vi "PID_controller_07.vi"() -> ()   [LabVIEW 2011]
uses:
  <vilib>/Platform/TimedLoop/XDataNode/nitl_modes.ctl
  <vilib>/Platform/TimedLoop/XDataNode/timing_clust.ctl
  <vilib>/Platform/TimedLoop/XDataNode/wakeup.ctl
  <vilib>/Platform/TimedLoop/XDataNode/XDataNode.xnode
  <vilib>/Platform/TimedLoop/XDataNode/XDNodeRunTimeDep.lvlib
panel:
  in  "Ks":dbl
  out "dt(s)":dbl
  out "windup error":dbl
  out "tPrev":dbl
  out "calc value":dbl
  out "error(t-t0)":cluster{dbl, "Value":dbl}[](array[cluster])
  out "error":dbl
  out "tStart(s)":dbl
  out "x-y":dbl
  out "S00":dbl
  out "S10":dbl
  out "S20":dbl
  out "S11":dbl
  out "S01":dbl
  out "weight":dbl[](array[numeric])
  in  "# of points to watch":i32
  in  "tSmooth(s)":dbl=-1.0
  out "t0":dbl
  out "error(t)":cluster{dbl, "Value":dbl}[](array[cluster])
  out "error out":errorcluster
  out "first":bool=TRUE
  out "P (torr)":string
  out "XY Graph":cluster{dbl, "Value":dbl}[](graph)
  out "current value":dbl
  in  "stop":bool
  in  "Period (s)":dbl
  out "dValue":dbl
  out "derivative":dbl
  out "integral":dbl
  out "Current angle (deg)":dbl
  in  "Kd":dbl
  in  "Ki":dbl
  in  "Kp":dbl
  out "Current P (torr)":dbl
  in  "Set Point (torr)":dbl
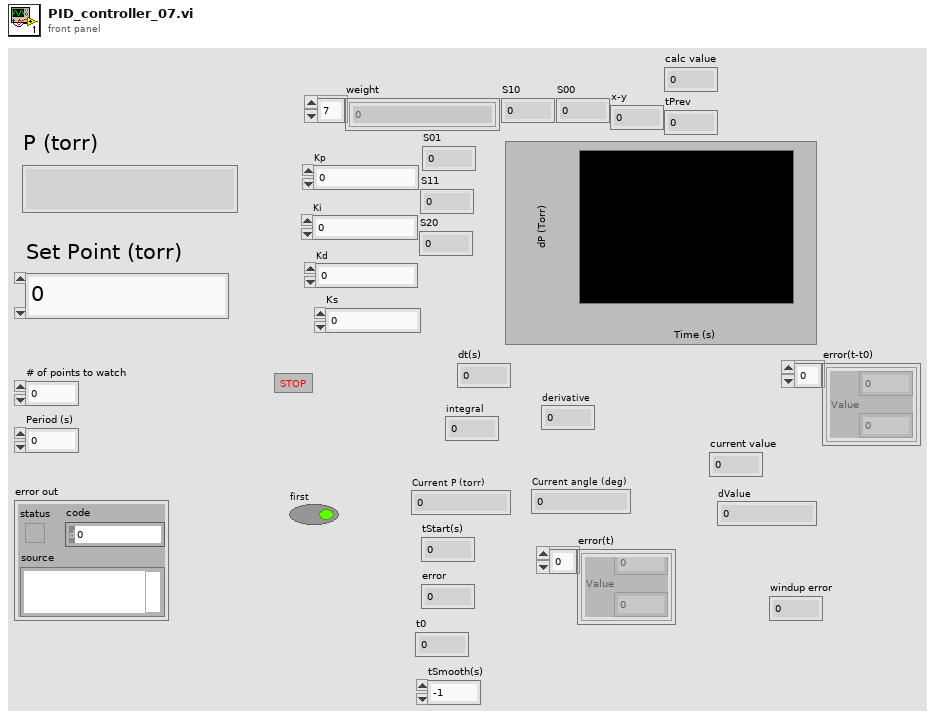
[diagram p1: front panel]
types:
  T1 = typedef "XDNodeRunTimeDep.lvlib/nitl_modes.ctl" = enum32{"No Change", "Process missed periods, maintain original phase", "Discard missed periods, maintain original phase", "Process missed periods, ignore original phase", "Discard missed periods, ignore original phase"}
  T2 = typedef "XDNodeRunTimeDep.lvlib/timing_clust.ctl" = cluster{"Expected End [f-1]":u64, "Actual End [f-1]":u64, "Finished Late? [f-1]":bool, "Expected End [i-1]":u64, "Actual End [i-1]":u64, "Finished Late? [i-1]":bool, "Expected Start [i]":u64, "Actual Start [i]":u64, "Expected Start [f]":u64, "Actual Start [f]":u64, "Source Name":string, "Structure Name":string, "Period":i64, "Deadline":i64, "Offset":i64, "Start":i64, "Priority":i32, "Timeout":i32, "Mode":T1, "Wakeup Reason":T3, "Error":errorcluster, "Source Type":string, "Secondary Source Type":string, "Global End Time":u64, "Global Start Time":u64, "Frame Duration":u64, "Iteration Duration":u64, "Assigned CPU":i32, "I/O Scan Engine Mode":u32}
  T3 = typedef "XDNodeRunTimeDep.lvlib/wakeup.ctl" = enum32{"Normal", "Aborted", "Asynchronous wakeup", "Timing source error", "Timed loop error", "Timeout"}
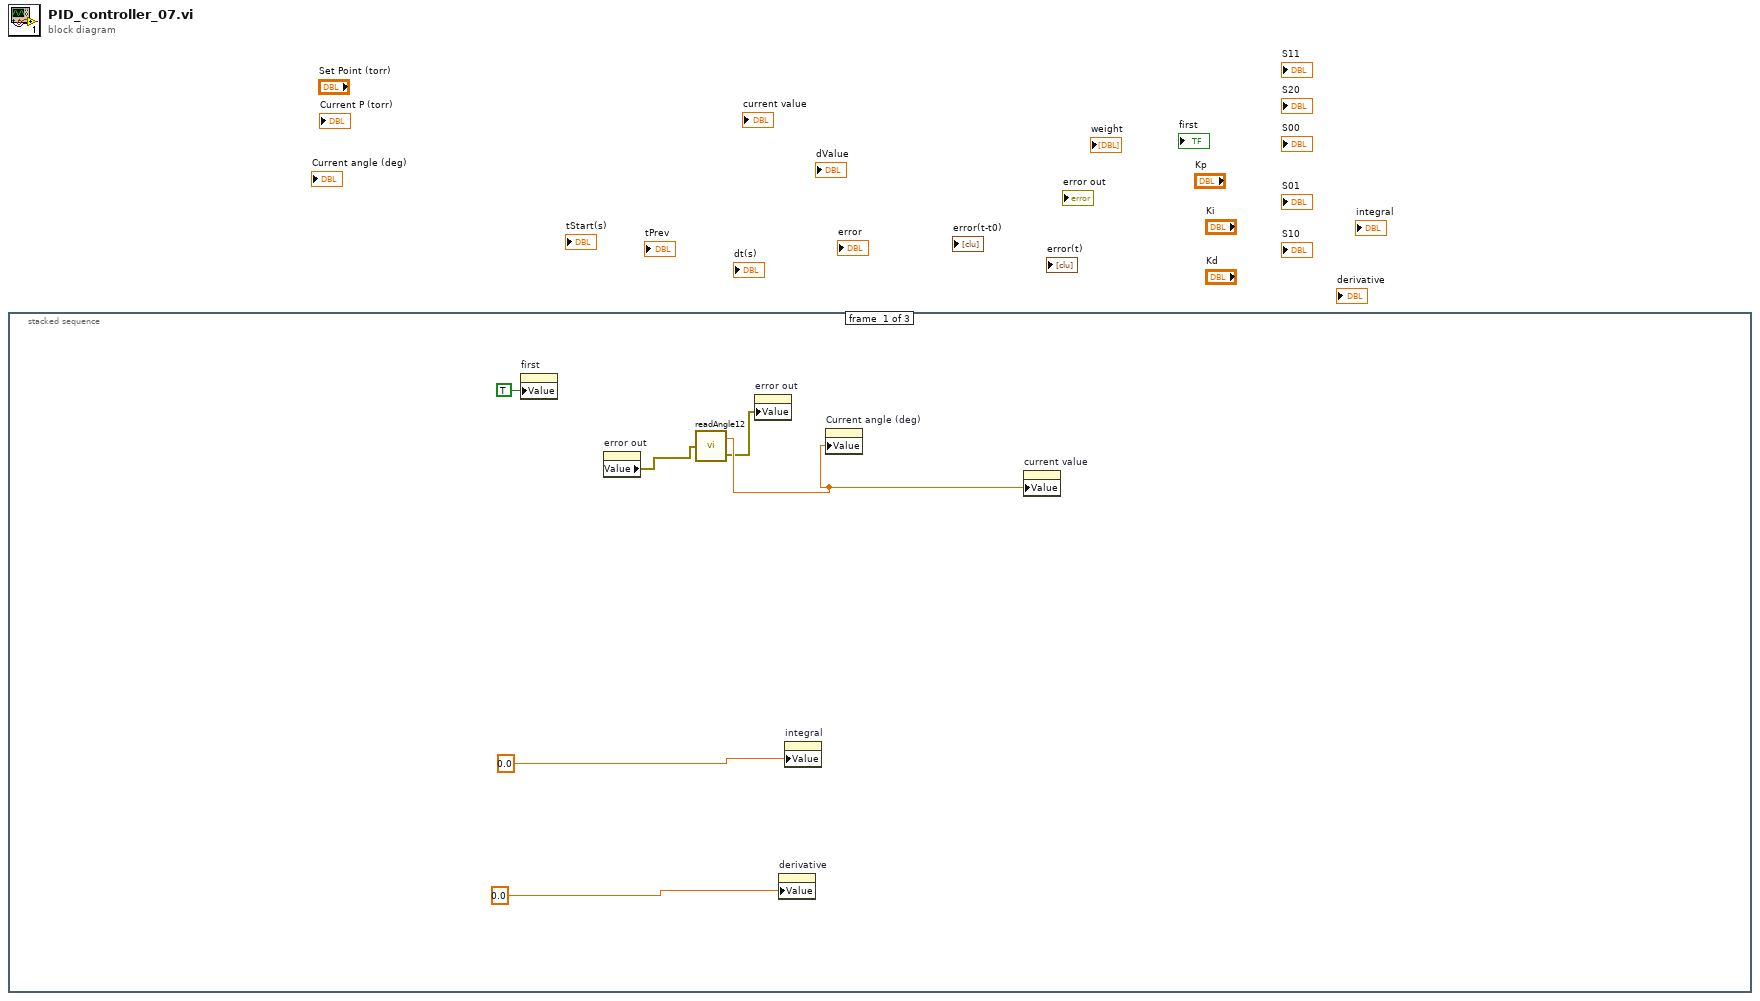
[diagram p0: block diagram]
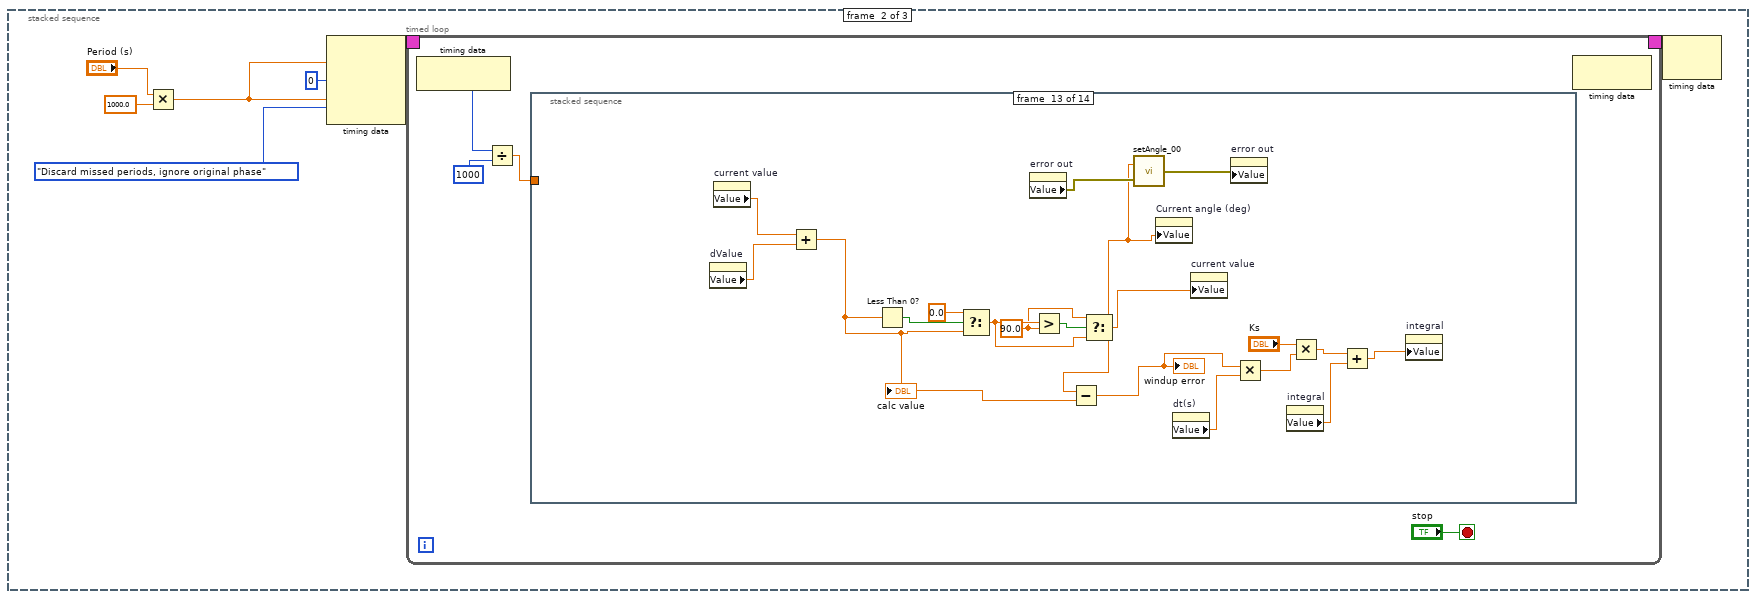
[diagram p2: hidden frame]
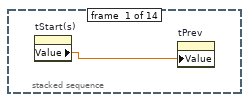
[diagram p3: hidden frame]
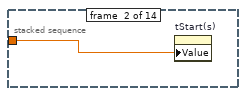
[diagram p4: hidden frame]
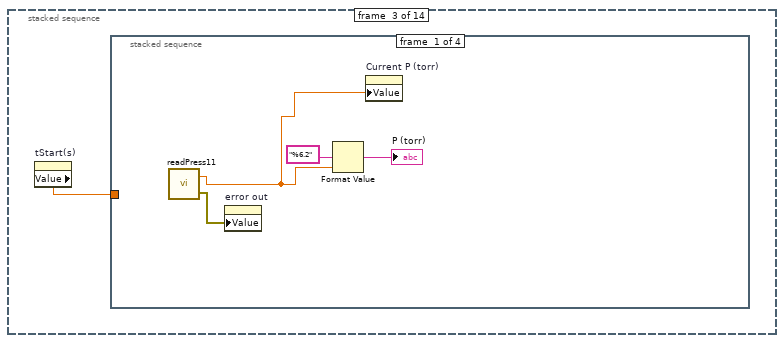
[diagram p5: hidden frame]
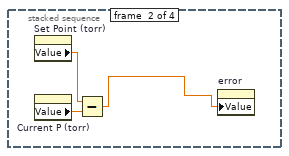
[diagram p6: hidden frame]
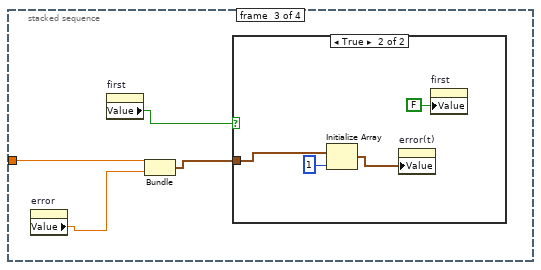
[diagram p7: hidden frame]
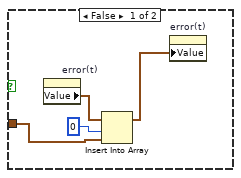
[diagram p8: hidden frame]
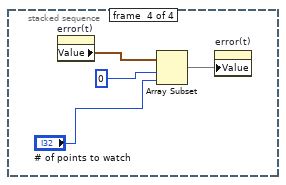
[diagram p9: hidden frame]
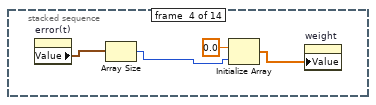
[diagram p10: hidden frame]
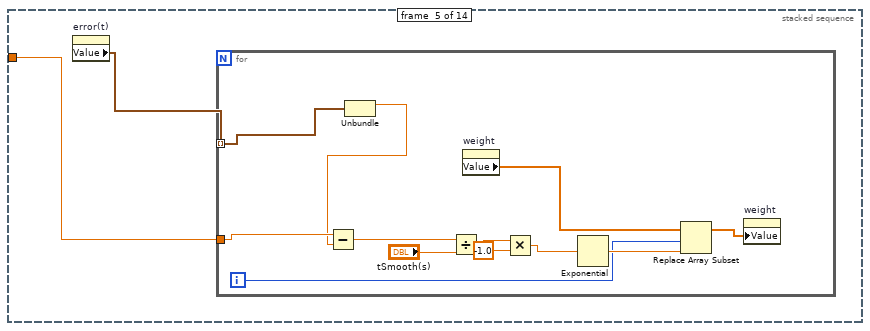
[diagram p11: hidden frame]
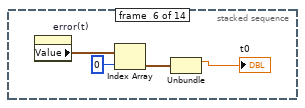
[diagram p12: hidden frame]
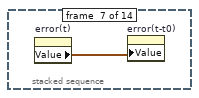
[diagram p13: hidden frame]
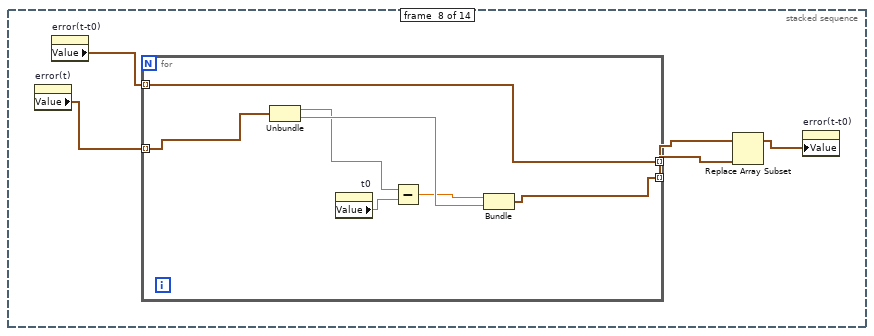
[diagram p14: hidden frame]
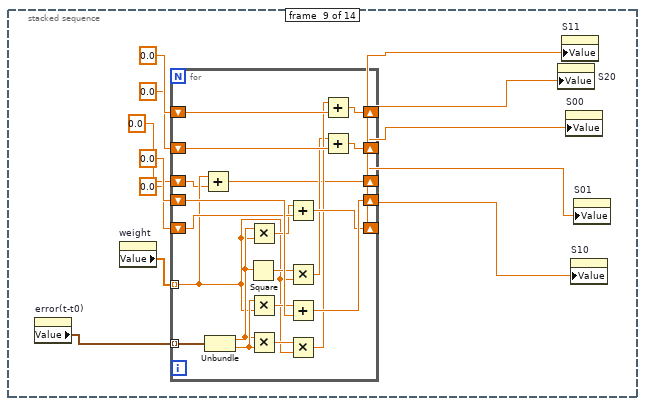
[diagram p15: hidden frame]
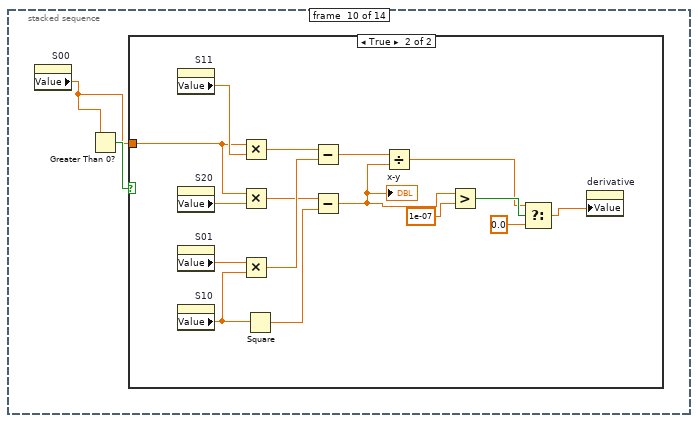
[diagram p16: hidden frame]
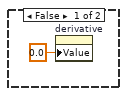
[diagram p17: hidden frame]
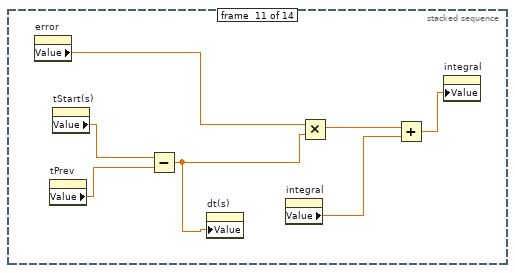
[diagram p18: hidden frame]
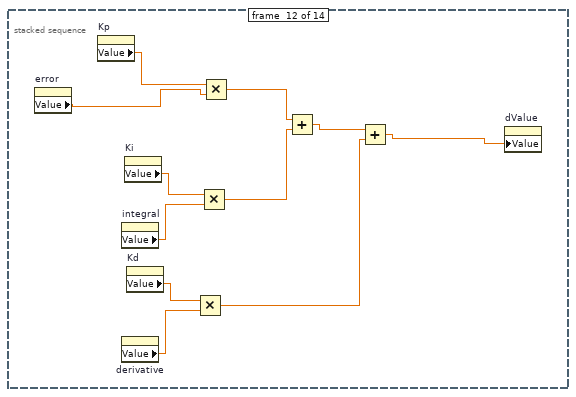
[diagram p19: hidden frame]
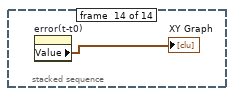
[diagram p20: hidden frame]
diagram:
  n1 = stacked-sequence {
    frame #0 {
      n2 = property on="first" class="Bool (strict)"("Value"=TRUE ("first")) -> ()  [unwired: 2 in, 2 out]
      n3 = property on="error out" class="Clust (strict)"() -> ("Value"=w2:errorcluster)  [unwired: 2 in, 2 out]
      n4 = call "readAngle12.vi"("error in"=w2) -> ("angle"=w3:dbl, "error out"=w1:errorcluster)
      n5 = property on="error out" class="Clust (strict)"("Value"=w1) -> ()  [unwired: 2 in, 2 out]
      n6 = property on="derivative" class="DigNum (strict)"("Value"=0.0 ("derivative")) -> ()  [unwired: 2 in, 2 out]
      n7 = property on="integral" class="DigNum (strict)"("Value"=0.0 ("integral")) -> ()  [unwired: 2 in, 2 out]
      n8 = property on="Current angle (deg)" class="DigNum (strict)"("Value"=w3) -> ()  [unwired: 2 in, 2 out]
      n9 = property on="current value" class="DigNum (strict)"("Value"=w3) -> ()  [unwired: 2 in, 2 out]
    }
    frame #1 {
      n10 = Multiply(x="Period (s)", y=1000.0) -> (x*y=w8:dbl)
      n11 = node-c288(w8, i64 0 ("Offset"), w8, nitl_modes."Discard missed periods, ignore original phase" ("Mode")) -> (w13:T2)
      n12 = timed-loop {
        timing: w13 -> [_]
        timing-out: [_] -> w12
        stop <- "stop" stop-if-true
        n13 = node-c288() -> (w14:i64)  [unwired: 1 in]
        n14 = Divide(x=w14, y=i64 1000) -> (x/y=w15:dbl)
        n15 = stacked-sequence {
          tunnel: w15 -> [_ w19 _ _ w48 _ _ _ _ _ _ _ _ _]
          frame #0 {
            n16 = property on="tStart(s)" class="DigNum (strict)"() -> ("Value"=w18:dbl)  [unwired: 2 in, 2 out]
            n17 = property on="tPrev" class="DigNum (strict)"("Value"=w18) -> ()  [unwired: 2 in, 2 out]
          }
          frame #1 {
            n18 = property on="tStart(s)" class="DigNum (strict)"("Value"=w19) -> ()  [unwired: 2 in, 2 out]
          }
          frame #2 {
            n19 = property on="tStart(s)" class="DigNum (strict)"() -> ("Value"=w20:dbl)  [unwired: 2 in, 2 out]
            n20 = stacked-sequence {
              tunnel: w20 -> [_ _ w30 _]
              frame #0 {
                n21 = call "readPress11.vi"() -> ("P"=w22:dbl, "error out"=w21:errorcluster)  [unwired: 1 in]
                n22 = property on="error out" class="Clust (strict)"("Value"=w21) -> ()  [unwired: 2 in, 2 out]
                n23 = Format Value(format string="%6.2", value (0)=w22) -> (output string=→"P (torr)":string)  [unwired: 1 in]
                n24 = property on="Current P (torr)" class="DigNum (strict)"("Value"=w22) -> ()  [unwired: 2 in, 2 out]
              }
              frame #1 {
                n25 = property on="Set Point (torr)" class="DigNum (strict)"() -> ("Value"=w26:dbl)  [unwired: 2 in, 2 out]
                n26 = property on="Current P (torr)" class="DigNum (strict)"() -> ("Value"=w27:dbl)  [unwired: 2 in, 2 out]
                n27 = Subtract(x=w26, y=w27) -> (x-y=w25:dbl)
                n28 = property on="error" class="DigNum (strict)"("Value"=w25) -> ()  [unwired: 2 in, 2 out]
              }
              frame #2 {
                n29 = property on="error" class="DigNum (strict)"() -> ("Value"=w28:dbl)  [unwired: 2 in, 2 out]
                n30 = property on="first" class="Bool (strict)"() -> ("Value"=w31:bool)  [unwired: 2 in, 2 out]
                n31 = Bundle("Value"=w30, "Value"=w28) -> (w29:cluster{"Value":dbl, "Value":dbl})  [unwired: 1 in]
                n32 = case shown="True" w31 {
                  tunnel: w29 -> [w33 w38]
                  frame False {
                    n33 = property on="error(t)" class="Arr (strict)"() -> ("Value"=w34:cluster{dbl, "Value":dbl}[])  [unwired: 2 in, 2 out]
                    n34 = Insert Into Array(array=w34, index=0, new element=w33) -> (w32:cluster{dbl, "Value":dbl}[])
                    n35 = property on="error(t)" class="Arr (strict)"("Value"=w32) -> ()  [unwired: 2 in, 2 out]
                  }
                  frame True {
                    n36 = Initialize Array(w38, 1 ("dimension size")) -> (w36:cluster{"Value":dbl, "Value":dbl}[])
                    n37 = property on="error(t)" class="Arr (strict)"("Value"=w36) -> ()  [unwired: 2 in, 2 out]
                    n38 = property on="first" class="Bool (strict)"("Value"=FALSE ("first")) -> ()  [unwired: 2 in, 2 out]
                  }
                }
              }
              frame #3 {
                n39 = property on="error(t)" class="Arr (strict)"() -> ("Value"=w41:cluster{dbl, "Value":dbl}[])  [unwired: 2 in, 2 out]
                n40 = Array Subset(array=w41, index=0, length="# of points to watch") -> (w43:cluster{dbl, "Value":dbl}[])
                n41 = property on="error(t)" class="Arr (strict)"("Value"=w43) -> ()  [unwired: 2 in, 2 out]
              }
            }
          }
          frame #3 {
            n42 = property on="error(t)" class="Arr (strict)"() -> ("Value"=w47:cluster{dbl, "Value":dbl}[])  [unwired: 2 in, 2 out]
            n43 = Array Size(array=w47) -> (size(s)=w45:i32)
            n44 = Initialize Array(0.0 ("element"), w45) -> (w44:dbl[])
            n45 = property on="weight" class="Arr (strict)"("Value"=w44) -> ()  [unwired: 2 in, 2 out]
          }
          frame #4 {
            n46 = property on="error(t)" class="Arr (strict)"() -> ("Value"=w49:cluster{dbl, "Value":dbl}[])  [unwired: 2 in, 2 out]
            n47 = for {
              tunnel: w49 -> [w61] mode=indexing
              tunnel: w48 -> [w60]
              i -> [w56]
              n48 = Unbundle(w61) -> (w59:dbl)  [unwired: 1 out]
              n49 = Subtract(x=w60, y=w59) -> (x-y=w54:dbl)
              n50 = Divide(x=w54, y="tSmooth(s)") -> (x/y=w52:dbl)
              n51 = property on="weight" class="Arr (strict)"() -> ("Value"=w57:dbl[])  [unwired: 2 in, 2 out]
              n52 = Multiply(x=w52, y=-1.0) -> (x*y=w50:dbl)
              n53 = Exponential(1:w50) -> (0:w58:dbl)
              n54 = Replace Array Subset(array=w57, new element=w58, index=w56) -> (w55:dbl[])
              n55 = property on="weight" class="Arr (strict)"("Value"=w55) -> ()  [unwired: 2 in, 2 out]
            }
          }
          frame #5 {
            n56 = property on="error(t)" class="Arr (strict)"() -> ("Value"=w65:cluster{dbl, "Value":dbl}[])  [unwired: 2 in, 2 out]
            n57 = Index Array(array=w65, index=0) -> (element=w63:cluster{dbl, "Value":dbl})
            n58 = Unbundle(w63) -> (→"t0":dbl)  [unwired: 1 out]
          }
          frame #6 {
            n59 = property on="error(t)" class="Arr (strict)"() -> ("Value"=w66:cluster{dbl, "Value":dbl}[])  [unwired: 2 in, 2 out]
            n60 = property on="error(t-t0)" class="Arr (strict)"("Value"=w66) -> ()  [unwired: 2 in, 2 out]
          }
          frame #7 {
            n61 = property on="error(t)" class="Arr (strict)"() -> ("Value"=w71:cluster{dbl, "Value":dbl}[])  [unwired: 2 in, 2 out]
            n62 = property on="error(t-t0)" class="Arr (strict)"() -> ("Value"=w69:cluster{dbl, "Value":dbl}[])  [unwired: 2 in, 2 out]
            n63 = for {
              tunnel: w71 -> [w74] mode=indexing
              tunnel: [w73] -> w70 mode=indexing
              tunnel: w69 -> [w72] mode=indexing
              tunnel: [w72] -> w68 mode=indexing
              n64 = Unbundle(w74) -> (w75:dbl, "Value"=w77:dbl)
              n65 = property on="t0" class="DigNum (strict)"() -> ("Value"=w78:dbl)  [unwired: 2 in, 2 out]
              n66 = Subtract(x=w75, y=w78) -> (x-y=w76:dbl)
              n67 = Bundle(w76, "Value"=w77) -> (w73:cluster{dbl, "Value":dbl})  [unwired: 1 in]
            }
            n68 = Replace Array Subset(array=w68, new element=w70) -> (w67:cluster{dbl, "Value":dbl}[])  [unwired: 1 in]
            n69 = property on="error(t-t0)" class="Arr (strict)"("Value"=w67) -> ()  [unwired: 2 in, 2 out]
          }
          frame #8 {
            n70 = property on="error(t-t0)" class="Arr (strict)"() -> ("Value"=w79:cluster{dbl, "Value":dbl}[])  [unwired: 2 in, 2 out]
            n71 = property on="weight" class="Arr (strict)"() -> ("Value"=w86:dbl[])  [unwired: 2 in, 2 out]
            n72 = for {
              tunnel: w79 -> [w106] mode=indexing
              shift-right: [w107] -> w81
              shift-left: 0.0 -> [w110]
              shift-right: [w103] -> w84
              shift-left: 0.0 -> [w109]
              shift-right: [w102] -> w83
              shift-left: 0.0 -> [w108]
              shift-right: [w104] -> w80
              shift-left: 0.0 -> [w105]
              tunnel: w86 -> [w93] mode=indexing
              shift-right: [w91] -> w82
              shift-left: 0.0 -> [w92]
              n73 = Add(x=w93, y=w92) -> (x+y=w91:dbl)
              n74 = Unbundle(w106) -> (w95:dbl, "Value"=w101:dbl)
              n75 = Square(x=w95) -> (x^2=w97:dbl)
              n76 = Multiply(x=w95, y=w93) -> (x*y=w94:dbl)
              n77 = Multiply(x=w101, y=w93) -> (x*y=w100:dbl)
              n78 = Multiply(x=w95, y=w101) -> (x*y=w99:dbl)
              n79 = Add(x=w94, y=w105) -> (x+y=w104:dbl)
              n80 = Multiply(x=w97, y=w93) -> (x*y=w96:dbl)
              n81 = Add(x=w100, y=w110) -> (x+y=w107:dbl)
              n82 = Multiply(x=w99, y=w93) -> (x*y=w98:dbl)
              n83 = Add(x=w98, y=w109) -> (x+y=w103:dbl)
              n84 = Add(x=w96, y=w108) -> (x+y=w102:dbl)
            }
            n85 = property on="S20" class="DigNum (strict)"("Value"=w83) -> ()  [unwired: 2 in, 2 out]
            n86 = property on="S11" class="DigNum (strict)"("Value"=w84) -> ()  [unwired: 2 in, 2 out]
            n87 = property on="S00" class="DigNum (strict)"("Value"=w82) -> ()  [unwired: 2 in, 2 out]
            n88 = property on="S10" class="DigNum (strict)"("Value"=w80) -> ()  [unwired: 2 in, 2 out]
            n89 = property on="S01" class="DigNum (strict)"("Value"=w81) -> ()  [unwired: 2 in, 2 out]
          }
          frame #9 {
            n90 = property on="S00" class="DigNum (strict)"() -> ("Value"=w111:dbl)  [unwired: 2 in, 2 out]
            n91 = Greater Than 0?(x=w111) -> (x > 0?=w112:bool)
            n92 = case shown="True" w112 {
              tunnel: w111 -> [_ w121]
              frame False {
                n93 = property on="derivative" class="DigNum (strict)"("Value"=0.0 ("derivative")) -> ()  [unwired: 2 in, 2 out]
              }
              frame True {
                n94 = property on="S11" class="DigNum (strict)"() -> ("Value"=w123:dbl)  [unwired: 2 in, 2 out]
                n95 = property on="S20" class="DigNum (strict)"() -> ("Value"=w122:dbl)  [unwired: 2 in, 2 out]
                n96 = property on="S01" class="DigNum (strict)"() -> ("Value"=w120:dbl)  [unwired: 2 in, 2 out]
                n97 = property on="S10" class="DigNum (strict)"() -> ("Value"=w124:dbl)  [unwired: 2 in, 2 out]
                n98 = Multiply(x=w121, y=w123) -> (x*y=w129:dbl)
                n99 = Multiply(x=w121, y=w122) -> (x*y=w127:dbl)
                n100 = Multiply(x=w120, y=w124) -> (x*y=w128:dbl)
                n101 = Square(x=w124) -> (x^2=w126:dbl)
                n102 = Subtract(x=w129, y=w128) -> (x-y=w125:dbl)
                n103 = Subtract(x=w127, y=w126) -> (x-y=w119:dbl)
                "x-y" <- w119
                n104 = Divide(x=w125, y=w119) -> (x/y=w115:dbl)
                n105 = Greater?(x=w119, y=1e-07) -> (0:w117:bool)
                n106 = Select(t=w115, s=w117, f=0.0) -> (s? t:f=w116:dbl)
                n107 = property on="derivative" class="DigNum (strict)"("Value"=w116) -> ()  [unwired: 2 in, 2 out]
              }
            }
          }
          frame #10 {
            n108 = property on="error" class="DigNum (strict)"() -> ("Value"=w134:dbl)  [unwired: 2 in, 2 out]
            n109 = property on="tPrev" class="DigNum (strict)"() -> ("Value"=w135:dbl)  [unwired: 2 in, 2 out]
            n110 = property on="tStart(s)" class="DigNum (strict)"() -> ("Value"=w136:dbl)  [unwired: 2 in, 2 out]
            n111 = Subtract(x=w136, y=w135) -> (x-y=w130:dbl)
            n112 = property on="dt(s)" class="DigNum (strict)"("Value"=w130) -> ()  [unwired: 2 in, 2 out]
            n113 = property on="integral" class="DigNum (strict)"() -> ("Value"=w132:dbl)  [unwired: 2 in, 2 out]
            n114 = Multiply(x=w134, y=w130) -> (x*y=w133:dbl)
            n115 = Add(x=w133, y=w132) -> (x+y=w131:dbl)
            n116 = property on="integral" class="DigNum (strict)"("Value"=w131) -> ()  [unwired: 2 in, 2 out]
          }
          frame #11 {
            n117 = property on="error" class="DigNum (strict)"() -> ("Value"=w137:dbl)  [unwired: 2 in, 2 out]
            n118 = property on="Kp" class="DigNum (strict)"() -> ("Value"=w147:dbl)  [unwired: 2 in, 2 out]
            n119 = property on="integral" class="DigNum (strict)"() -> ("Value"=w145:dbl)  [unwired: 2 in, 2 out]
            n120 = property on="derivative" class="DigNum (strict)"() -> ("Value"=w143:dbl)  [unwired: 2 in, 2 out]
            n121 = property on="Ki" class="DigNum (strict)"() -> ("Value"=w146:dbl)  [unwired: 2 in, 2 out]
            n122 = property on="Kd" class="DigNum (strict)"() -> ("Value"=w144:dbl)  [unwired: 2 in, 2 out]
            n123 = Multiply(x=w144, y=w143) -> (x*y=w140:dbl)
            n124 = Multiply(x=w146, y=w145) -> (x*y=w141:dbl)
            n125 = Multiply(x=w147, y=w137) -> (x*y=w142:dbl)
            n126 = Add(x=w142, y=w141) -> (x+y=w139:dbl)
            n127 = Add(x=w139, y=w140) -> (x+y=w138:dbl)
            n128 = property on="dValue" class="DigNum (strict)"("Value"=w138) -> ()  [unwired: 2 in, 2 out]
          }
          frame #12 {
            w157 = 90.0 ("y")
            n129 = property on="dValue" class="DigNum (strict)"() -> ("Value"=w164:dbl)  [unwired: 2 in, 2 out]
            n130 = property on="current value" class="DigNum (strict)"() -> ("Value"=w165:dbl)  [unwired: 2 in, 2 out]
            n131 = Add(x=w165, y=w164) -> (x+y=w148:dbl)
            "calc value" <- w148
            n132 = Less Than 0?(x=w148) -> (x < 0?=w161:bool)
            n133 = Select(t=0.0, s=w161, f=w148) -> (s? t:f=w158:dbl)
            n134 = property on="error out" class="Clust (strict)"() -> ("Value"=w163:errorcluster)  [unwired: 2 in, 2 out]
            n135 = Greater?(x=w158, y=w157) -> (0:w159:bool)
            n136 = Select(t=w157, s=w159, f=w158) -> (s? t:f=w149:dbl)
            n137 = Subtract(x=w149, y=w148) -> (x-y=w156:dbl)
            "windup error" <- w156
            n138 = call "setAngle_00.vi"("error in (no error)"=w163, "Angle (deg)"=w149) -> ("error out"=w162:errorcluster)
            n139 = property on="Current angle (deg)" class="DigNum (strict)"("Value"=w149) -> ()  [unwired: 2 in, 2 out]
            n140 = property on="dt(s)" class="DigNum (strict)"() -> ("Value"=w155:dbl)  [unwired: 2 in, 2 out]
            n141 = property on="current value" class="DigNum (strict)"("Value"=w149) -> ()  [unwired: 2 in, 2 out]
            n142 = property on="error out" class="Clust (strict)"("Value"=w162) -> ()  [unwired: 2 in, 2 out]
            n143 = Multiply(x=w156, y=w155) -> (x*y=w154:dbl)
            n144 = property on="integral" class="DigNum (strict)"() -> ("Value"=w151:dbl)  [unwired: 2 in, 2 out]
            n145 = Multiply(x="Ks", y=w154) -> (x*y=w152:dbl)
            n146 = Add(x=w152, y=w151) -> (x+y=w150:dbl)
            n147 = property on="integral" class="DigNum (strict)"("Value"=w150) -> ()  [unwired: 2 in, 2 out]
          }
          frame #13 {
            n148 = property on="error(t-t0)" class="Arr (strict)"() -> ("Value"=→"XY Graph":cluster{dbl, "Value":dbl}[])  [unwired: 2 in, 2 out]
          }
        }
        n149 = node-c288() -> ()  [unwired: 1 in, 1 out]
      }
      n150 = node-c288(w12) -> ()  [unwired: 1 out]
    }
    frame #2 {
      n151 = call "WriteAdaptorr03.vi"("string to write"="D5") -> ()  [unwired: 1 in, 1 out]
    }
  }
